vi "Main.vi"(11 "Module Admin":refnum<class "Delacor_lib_QMH_Module Admin.lvclass">) -> ()   [LabVIEW 2023, in "TDMS.lvlib"]
doc: "This template is based off of the Queued Message Handler design pattern and the Queued Message Handler project template that ships with LabVIEW.\n\nThe main difference is that the queue is private to this module and communication between modules is performed via Broadcast and Request events.\n\nRequest events are wrapped in public API methods and are handled in the Event Handling Loop (EHL) of this VI. Any module can register for Broadcast events sent by this module. The EHL generates messages based on user interface actions.\n\nThe Message Handling Loop (MHL) processes messages generated by the EHL, or by other messages. The messages are string values, so new messages can be added easily to the Message Cases case structure in the MHL. Each message cluster can also provide an optional value for Message Data, which is a variant that can be converted to whatever message-specific data is required.\n_____\nBased on DQMH Project Template 7.0.1.1316."
uses:
  TDMS.lvlib
  <vilib>/Delacor/Delacor QMH/Libraries/Module Admin_class/Delacor_lib_QMH_Module Admin.lvclass
  Module Data--cluster.ctl
  Stop Argument--cluster.ctl
  <vilib>/Delacor/Delacor QMH/Libraries/Message Queue_class/Delacor_lib_QMH_Message Queue.lvclass/Delacor_lib_QMH_Message Queue.ctl
  <vilib>/Delacor/Delacor QMH/Libraries/Module Admin_class/Delacor_lib_QMH_Module Admin.lvclass/Delacor_lib_QMH_Module Admin.ctl
  Write Data Argument--cluster.ctl
  Libraries/RT Main/Data Cluster.ctl
  <vilib>/Delacor/Delacor QMH/Libraries/Message Queue_class/Delacor_lib_QMH_Enqueue Message (Single).vi
  <vilib>/Delacor/Delacor QMH/Libraries/Module Admin_class/Delacor_lib_QMH_Get External Launch.vi
  <vilib>/Delacor/Delacor QMH/Libraries/Message Queue_class/Delacor_lib_QMH_Message Queue.lvclass
  Libraries/RT Main/RT Main.lvlib
  <vilib>/WebDAVClient/NI_WebDAV.lvlib
  <vilib>/WebDAVClient/Advanced/Get File.vi
panel:
  out "error out":errorcluster
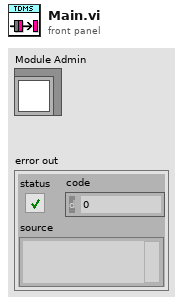
[diagram p1: front panel]
types:
  T1 = typedef "TDMS.lvlib/Request Events--cluster.ctl" = cluster{"Stop Module":refnum<user-event>, "Show Panel":refnum<user-event>, "Hide Panel":refnum<user-event>, "Get Module Execution Status":refnum<user-event>, "Show Diagram":refnum<user-event>, "Create TDMS File":refnum<user-event>, "Close TDMS File":refnum<user-event>, "Write Data":refnum<user-event>, "Private.Write Data to File":refnum<user-event>}
  T2 = typedef "TDMS.lvlib/Module Data--cluster.ctl" = cluster{"Status":string, "Path":path, "tdms file Ref":refnum<k34>}
  T3 = enum32{"invalid lock state", "Not Locked", "Locked (No Password)", "Password-protected"}
  T4 = typedef "TDMS.lvlib/Stop Argument--cluster.ctl" = cluster{"Origin":string, "Exit via Stop Module Req?":bool, "Wait for Module to stop?":bool}
  T5 = typedef "TDMS.lvlib/Write Data Argument--cluster.ctl" = cluster{"Data":T6[]}
  T6 = typedef "RT Main.lvlib/Data Cluster.ctl" = cluster{"Analog Input":dbl[], "Digital Inputs":bool[], "U32":u32[]}
  T7 = enum16{"open", "open or create", "create or replace", "create", "open (read-only)"}
  T8 = typedef "NI_WebDAV.lvlib/SessionHandle.ctl" = refnum<k1>
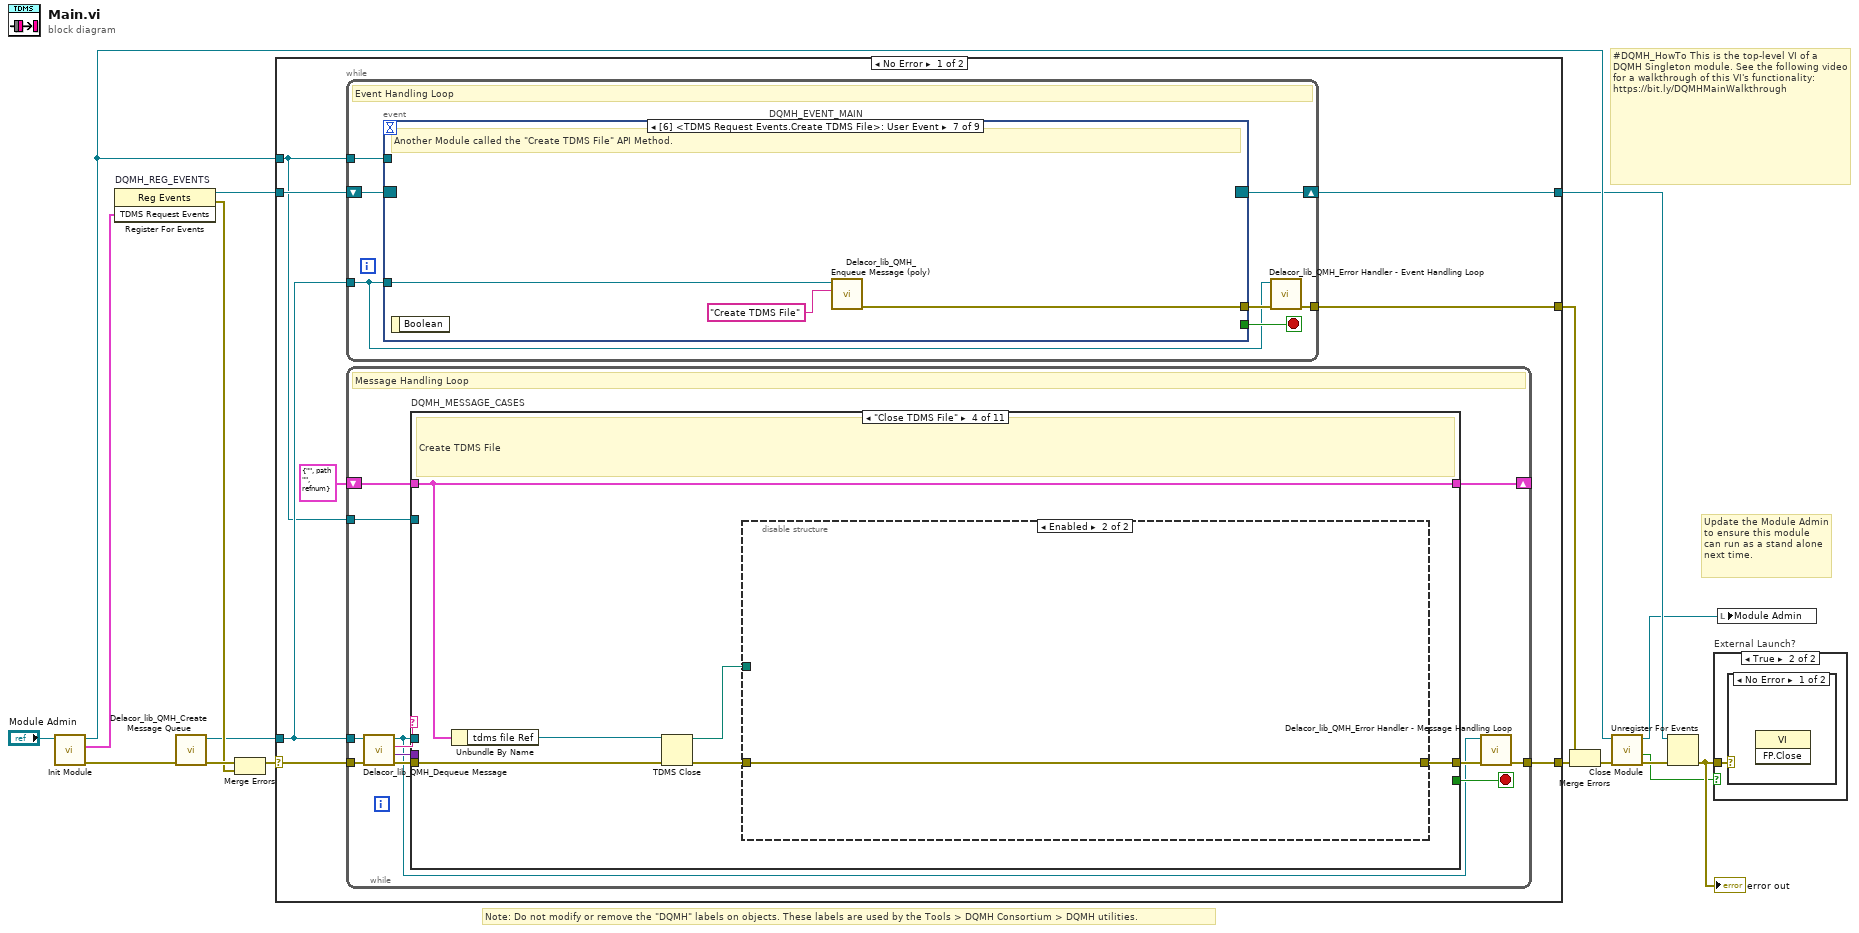
[diagram p0: block diagram]
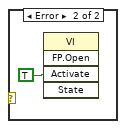
[diagram p3: hidden frame]
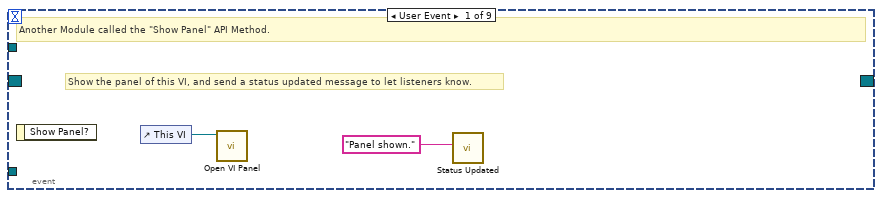
[diagram p4: hidden frame]
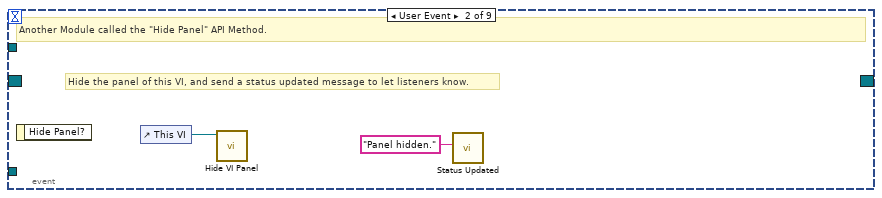
[diagram p5: hidden frame]
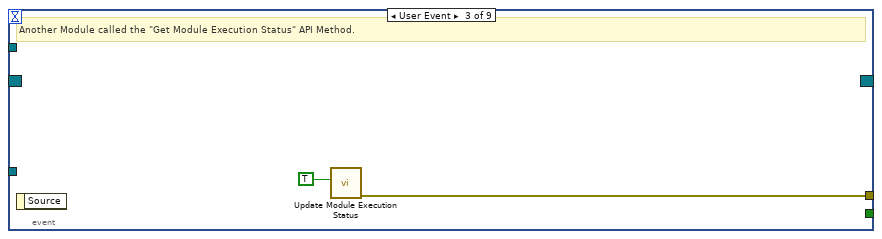
[diagram p6: hidden frame]
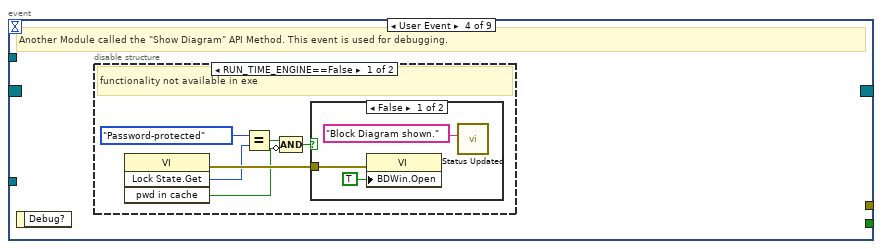
[diagram p7: hidden frame]
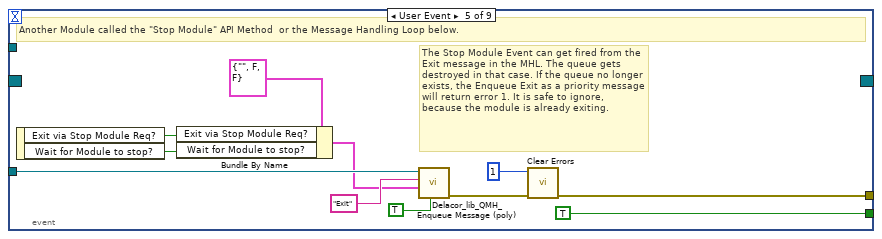
[diagram p10: hidden frame]
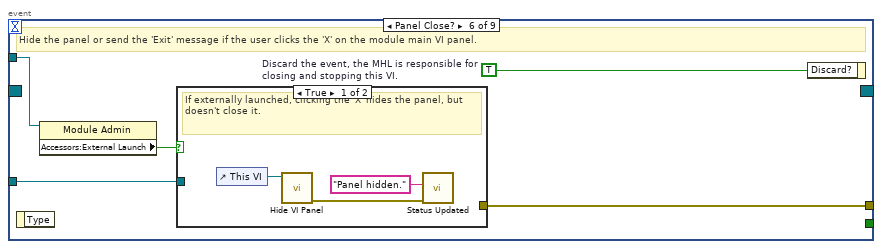
[diagram p11: hidden frame]
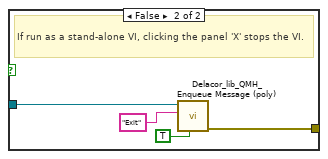
[diagram p12: hidden frame]
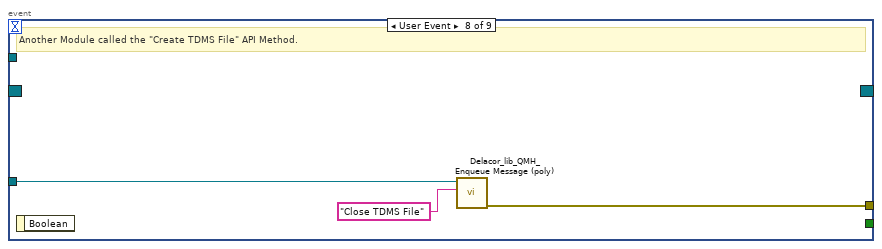
[diagram p13: hidden frame]
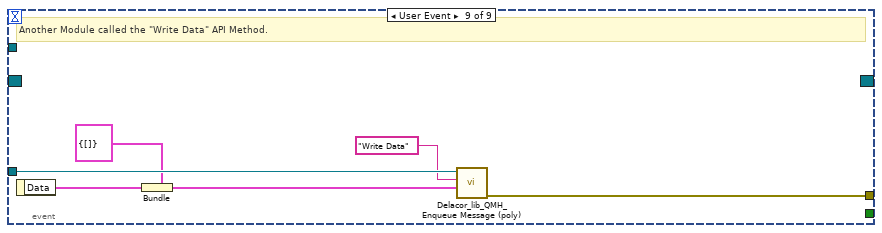
[diagram p14: hidden frame]
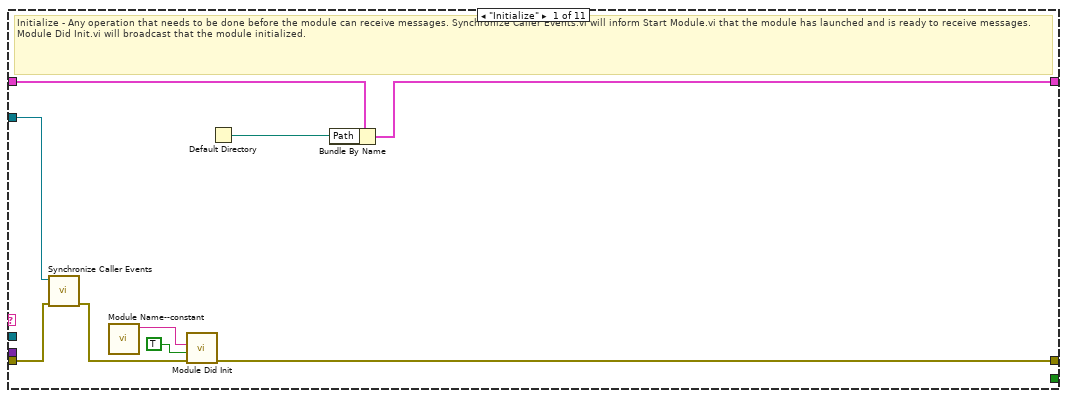
[diagram p15: hidden frame]
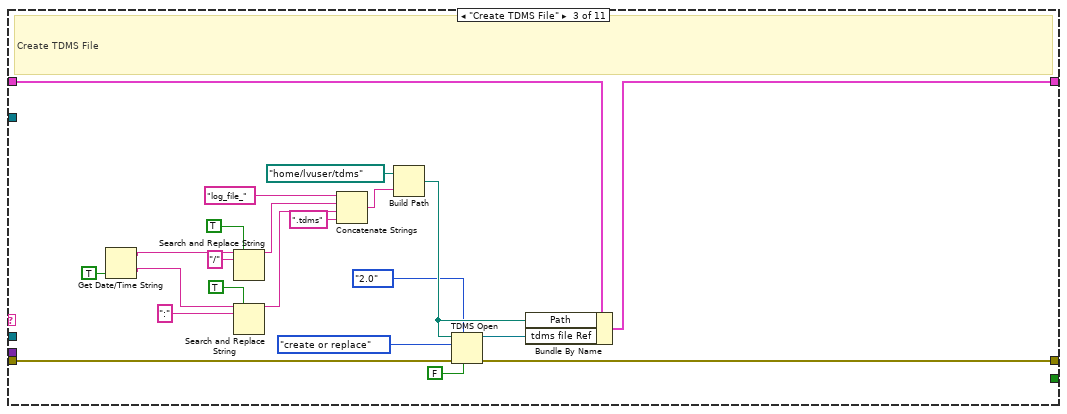
[diagram p17: hidden frame]
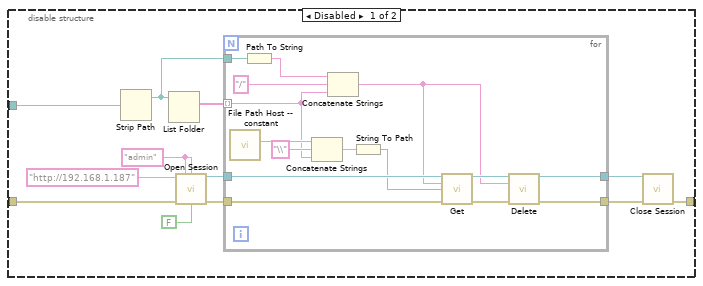
[diagram p18: hidden frame]
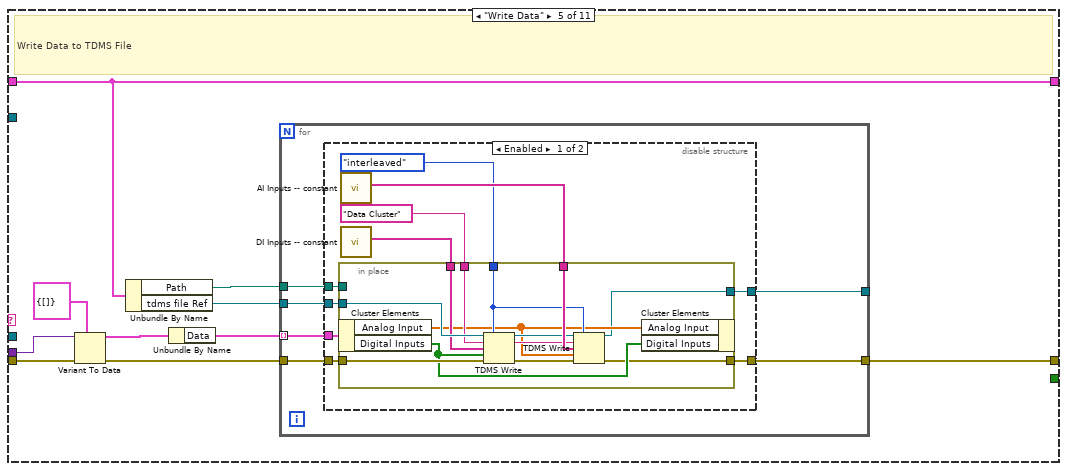
[diagram p19: hidden frame]
diagram:
  # "#DQMH_HowTo This is the top-level VI of a DQMH Singleton module. See the following video for a walkthrough of this VI's functionality: https://bit.ly/DQMHMainWalkthrough"
  # "Note: Do not modify or remove the \"DQMH\" labels on objects. These labels are used by the Tools > DQMH Consortium > DQMH utilities."
  # "Update the Module Admin to ensure this module can run as a stand alone next time."
  n1 = call "Init Module.vi"("Singleton Module Admin in"="Module Admin") -> ("error out"=w16:errorcluster, "TDMS Request Events"=w1:T1, "Singleton Module Admin out"=w8:refnum<class "Delacor_lib_QMH_Module Admin.lvclass">)  [unwired: 8 in]
  n2 = register-events "DQMH_REG_EVENTS"(w1) -> (reference out=w6:refnum<event-registration>, error out=w9:errorcluster)  [unwired: 2 in]
  n3 = call <vilib>:"Delacor_lib_QMH_Create Message Queue.vi"("error in"=w16) -> ("error out"=w11:errorcluster, "Message Queue"=w5:refnum<class "Delacor_lib_QMH_Message Queue.lvclass">)  [unwired: 9 in]
  n4 = Merge Errors(w11, w9) -> (w10:errorcluster)
  n5 = case shown="No Error" w10 {
    selector: w10 -> [w23 w265]
    tunnel: [w25 w264] -> w17
    tunnel: [w22 w263] -> w7
    tunnel: w6 -> [w20 w263]
    tunnel: w5 -> [w19 w258]
    tunnel: [w24 _] -> w14
    tunnel: w8 -> [w18 w259]
    frame No Error {
      n6 = while {
        tunnel: w19 -> [w26]
        shift-right: [w29] -> w22
        shift-left: w20 -> [w30]
        tunnel: [w31] -> w24
        tunnel: w18 -> [w27]
        stop <- w28 stop-if-true
        # "Event Handling Loop"
        n7 = event "DQMH_EVENT_MAIN" shown="[6] <TDMS Request Events.Create TDMS File>: User Event" {
          selector: w30 -> [_ _ _ _ _ _ _ _ _]
          dyn-events: [_ _ _ _ _ _ _ _ _] -> w29
          timeout: _ -> [_ _ _ _ _ _ _ _ _]
          tunnel: [_ _ _ _ TRUE ("Discard?") _ _ _ _] -> w28
          tunnel: w26 -> [_ _ _ _ w54 w61 w73 w76 w82]
          tunnel: [_ _ w38 _ w57 w63 w71 w74 w77] -> w32
          tunnel: w27 -> [_ _ _ _ _ w60 _ _ _]
          event User Event {
            # "Show the panel of this VI, and send a status updated message to let listeners know."
            # "Another Module called the \"Show Panel\" API Method."
            n8 = event-data() -> ()  [unwired: 1 in, 1 out]
            n9 = control-ref of="This VI"() -> (w34:refnum<vi>)
            n10 = call "Open VI Panel.vi"("VI"=w34) -> ()  [unwired: 10 in, 1 out]
            n11 = call "Status Updated.vi"("Status"="Panel shown." ("format string")) -> ()  [unwired: 10 in, 1 out]
          }
          event User Event {
            # "Hide the panel of this VI, and send a status updated message to let listeners know."
            # "Another Module called the \"Hide Panel\" API Method."
            n12 = event-data() -> ()  [unwired: 1 in, 1 out]
            n13 = control-ref of="This VI"() -> (w36:refnum<vi>)
            n14 = call "Hide VI Panel.vi"("VI"=w36) -> ()  [unwired: 10 in, 1 out]
            n15 = call "Status Updated.vi"("Status"="Panel hidden." ("format string")) -> ()  [unwired: 10 in, 1 out]
          }
          event User Event {
            # "Another Module called the \"Get Module Execution Status\" API Method."
            n16 = event-data() -> ()  [unwired: 1 in, 1 out]
            n17 = call "Update Module Execution Status.vi"("Running?"=TRUE) -> ("error out"=w38:errorcluster)  [unwired: 10 in]
          }
          event User Event {
            # "Another Module called the \"Show Diagram\" API Method. This event is used for debugging."
            n18 = event-data() -> ()  [unwired: 1 in, 1 out]
            n19 = disable-structure shown="RUN_TIME_ENGINE==False" {
              frame condition #0 (active) {
                # "functionality not available in exe"
                n20 = invoke on="Invoke Node" class="VI" method="Lock State.Get"() -> (error out=w44:errorcluster, "Get Lock State"=w43:T3, "pwd in cache"=w40:bool)  [unwired: 4 in, 1 out]
                n21 = Equal?(x=T3."Password-protected", y=w43) -> (x = y?=w41:bool)
                n22 = Compound Arithmetic op=AND(w41, invert w40) -> (w39:bool)
                n23 = case shown="False" w39 {
                  tunnel: w44 -> [w47 _]
                  frame False {
                    n24 = property on="Property Node" class="VI"(error in=w47, "BDWin.Open"=TRUE ("Block Diagram Window:Open")) -> ()  [unwired: 1 in, 2 out]
                    n25 = call "Status Updated.vi"("Status"="Block Diagram shown." ("format string")) -> ()  [unwired: 10 in, 1 out]
                  }
                  frame True {
                    # "Password-protected VI, and the password is not in the cache. Do not show the diagram."
                  }
                }
              }
              frame condition #1 {
              }
            }
          }
          event User Event {
            # "The Stop Module Event can get fired from the Exit message in the MHL. The queue gets destroyed in that case. If the queue no longer exists, the Enqueue Exit as a priority message will return error 1. It is safe to ignore, because the module is already exiting."
            # "Another Module called the \"Stop Module\" API Method  or the Message Handling Loop below."
            n26 = event-data() -> ("Exit via Stop Module Req?"=w50:bool, "Wait for Module to stop?"=w49:bool)  [unwired: 1 in]
            n27 = Bundle By Name(cluster=T4 {"Origin"="", "Exit via Stop Module Req?"=FALSE, "Wait for Module to stop?"=FALSE} ("Stop Argument"), "Exit via Stop Module Req?"=w50, "Wait for Module to stop?"=w49) -> (w48:T4)
            n28 = call-poly <vilib>:"Delacor_lib_QMH_Enqueue Message (poly).vi"("Priority Message? (F)"=TRUE, "Message Data"=w48, "Message"="Exit", "Message Queue in"=w54) -> ("error out"=w58:errorcluster)  [unwired: 6 in, 1 out]
            n29 = call <vilib>:"Clear Errors.vi"("error in (no error)"=w58, "specific error code to clear (0: all)"=1) -> ("error out"=w57:errorcluster)  [unwired: 4 in, 1 out]
          }
          event Panel Close? {
            w62 = TRUE  # Discard the event, the MHL is responsible for closing and stopping this VI.
            # "Hide the panel or send the 'Exit' message if the user clicks the 'X' on the module main VI panel."
            n30 = event-data() -> ()  [unwired: 1 in, 1 out]
            n31 = property on="Property Node" class="Module Admin"(reference=w60) -> ("Accessors:External Launch"=w59:bool)  [unwired: 1 in, 2 out]
            n32 = case shown="True" w59 {
              tunnel: w61 -> [_ w69]
              tunnel: [_ w70] -> w63
              frame True {
                # "If externally launched, clicking the 'X' hides the panel, but doesn't close it."
                n33 = control-ref of="This VI"() -> (w66:refnum<vi>)
                n34 = call "Hide VI Panel.vi"("VI"=w66) -> ("error out"=w64:errorcluster)  [unwired: 10 in]
                n35 = call "Status Updated.vi"("error in"=w64, "Status"="Panel hidden." ("format string")) -> ()  [unwired: 9 in, 1 out]
              }
              frame False {
                # "If run as a stand-alone VI, clicking the panel 'X' stops the VI."
                n36 = call-poly <vilib>:"Delacor_lib_QMH_Enqueue Message (poly).vi"("Priority Message? (F)"=TRUE, "Message"="Exit", "Message Queue in"=w69) -> ("error out"=w70:errorcluster)  [unwired: 7 in, 1 out]
              }
            }
            n37 = event-data ("Event Filter Node")("Discard?"=w62) -> ()  [unwired: 1 in, 1 out]
          }
          event User Event {
            # "Another Module called the \"Create TDMS File\" API Method."
            n38 = event-data() -> ()  [unwired: 1 in, 1 out]
            n39 = call-poly <vilib>:"Delacor_lib_QMH_Enqueue Message (poly).vi"("Message"="Create TDMS File", "Message Queue in"=w73) -> ("error out"=w71:errorcluster)  [unwired: 8 in, 1 out]
          }
          event User Event {
            # "Another Module called the \"Create TDMS File\" API Method."
            n40 = event-data() -> ()  [unwired: 1 in, 1 out]
            n41 = call-poly <vilib>:"Delacor_lib_QMH_Enqueue Message (poly).vi"("Message"="Close TDMS File", "Message Queue in"=w76) -> ("error out"=w74:errorcluster)  [unwired: 8 in, 1 out]
          }
          event User Event {
            # "Another Module called the \"Write Data\" API Method."
            n42 = event-data() -> ("Data"=w78:T6[])  [unwired: 1 in]
            n43 = Bundle(cluster=T5 {"Data"=[]} ("Write Data Argument"), "Data"=w78) -> (w79:T5)
            n44 = call-poly <vilib>:"Delacor_lib_QMH_Enqueue Message (poly).vi"("Message Data"=w79, "Message"="Write Data", "Message Queue in"=w82) -> ("error out"=w77:errorcluster)  [unwired: 7 in, 1 out]
          }
        }
        n45 = call-dynamic "Delacor_lib_QMH_Error Handler - Event Handling Loop.vi"("error in"=w32, "Message Queue in"=w26) -> ("dup error in"=w31:errorcluster)  [unwired: 8 in, 1 out]
      }
      n46 = while {
        tunnel: w19 -> [w83]
        shift-right: [w91] -> _
        shift-left: T2 {"Status"="", "Path"=path "", "tdms file Ref"=refnum} ("Data Cluster") -> [w92]
        tunnel: w23 -> [w94]
        tunnel: [w86] -> w25
        tunnel: w18 -> [w87]
        stop <- w90 stop-if-true
        # "Message Handling Loop"
        n47 = call-dynamic "Delacor_lib_QMH_Dequeue Message.vi"("error in"=w94, "Message Queue in"=w83) -> ("error out"=w93:errorcluster, "Message Data"=w88:variant, "Message"=w89:string, "Message Queue out"=w84:refnum<class "Delacor_lib_QMH_Message Queue.lvclass">)  [unwired: 6 in]
        n48 = case "DQMH_MESSAGE_CASES" shown="\"Close TDMS File\"" w89 {
          selector: w89 -> [_ _ _ _ _ _ _ _ _ _ w253]
          tunnel: w84 -> [_ _ _ _ _ _ _ _ w219 w241 _]
          tunnel: w93 -> [w103 w105 w126 w128 w171 w204 w206 w215 w226 w247 w256]
          tunnel: [w98 w105 w127 w130 w162 w203 w206 w214 w222 w242 w257] -> w85
          tunnel: w92 -> [w96 w104 w111 w133 w166 w202 w205 w212 w221 w240 w254]
          tunnel: [w97 w104 w112 w133 w166 w202 w205 w212 w221 w240 w254] -> w91
          tunnel: [_ _ _ _ _ _ _ _ _ w239 _] -> w90
          tunnel: w88 -> [_ _ _ _ w170 _ _ _ w220 w238 _]
          tunnel: w87 -> [w101 _ _ _ _ _ _ _ w218 w233 _]
          frame "Initialize" {
            # "Initialize - Any operation that needs to be done before the module can receive messages. Synchronize Caller Events.vi will inform Start Module.vi that the module has launched and is ready to receive messages. Module Did Init.vi will broadcast that the module initialized."
            n49 = call "Synchronize Caller Events.vi"("error in"=w103, "Singleton Module Admin in"=w101) -> ("error out"=w102:errorcluster)  [unwired: 8 in, 1 out]
            n50 = call "Module Name--constant.vi"() -> ("Module Name"=w99:string)  [unwired: 11 in]
            n51 = call "Module Did Init.vi"("error in"=w102, "Initialized?"=TRUE, "Origin"=w99) -> ("error out"=w98:errorcluster)  [unwired: 8 in]
            n52 = Default Directory() -> (w95:path)
            n53 = Bundle By Name(cluster=w96, "Path"=w95) -> (w97:T2)
          }
          frame "---Module Specific---" {
            # "Separator -- The following cases handle messages specific to this Module."
          }
          frame "Create TDMS File" {
            # "Create TDMS File"
            n54 = Get Date/Time String(want seconds? (F)=TRUE) -> (date string=w118:string, time string=w117:string)  [unwired: 2 in]
            n55 = Search and Replace String(replace all?=TRUE ("replace all? (F)"), input string=w118, search string="/") -> (result string=w116:string)  [unwired: 5 in, 3 out]
            n56 = Search and Replace String(replace all?=TRUE ("replace all? (F)"), input string=w117, search string=":") -> (result string=w115:string)  [unwired: 5 in, 3 out]
            n57 = Concatenate Strings("log_file_", w116, w115, ".tdms" ("string")) -> (w113:string)
            n58 = Build Path(base path=path "/home/lvuser/tdms", name or relative path=w113) -> (appended path=w108:path)
            n59 = TDMS Open(6:FALSE ("disable buffering? (T)"), 7:enum16{"1.0", "2.0"}."2.0" ("file format version (2.0)"), 8:w126, 10:T7."create or replace" ("operation (0:open)"), 11:w108) -> (0:w127:errorcluster, 3:w125:refnum<k34>)  [unwired: 2 in]
            n60 = Bundle By Name(cluster=w111, "Path"=w108, "tdms file Ref"=w125) -> (w112:T2)
          }
          frame "Close TDMS File" {
            # "Create TDMS File"
            n61 = Unbundle By Name(w133) -> ("tdms file Ref"=w129:refnum<k34>)
            n62 = TDMS Close(8:w128, 11:w129) -> (0:w131:errorcluster, 3:w132:path)
            n63 = disable-structure shown="Enabled" {
              disable-tunnel: w132 -> [w145 _]
              disable-tunnel: w131 -> [w143 w161]
              disable-tunnel: [w134 w161] -> w130
              frame Disabled {
                w140 = "admin" ("username")
                n64 = Strip Path(path=w145) -> (stripped path=w137:path)  [unwired: 1 out]
                n65 = List Folder(path=w137) -> (filenames=w144:string[])  [unwired: 3 in, 3 out]
                n66 = call <vilib>:"Open Session.vi"("host uri prefix"="http://192.168.1.187", "username"=w140, "password"=w140, "error in (no error)"=w143, "verify server?"=FALSE) -> ("session handle out"=w141:T8, "error out"=w142:errorcluster)  [unwired: 9 in]
                n67 = for {
                  tunnel: w144 -> [w148] mode=indexing
                  tunnel: w142 -> [w156]
                  tunnel: w141 -> [w160]
                  tunnel: w137 -> [w159]
                  tunnel: [w152] -> w136
                  tunnel: [w151] -> w135
                  n68 = call "File Path Host -- constant.vi"() -> ("File Path Control"=w150:string)  [unwired: 11 in]
                  n69 = Path To String(path=w159) -> (string=w158:string)
                  n70 = Concatenate Strings(w150, "\\" ("string"), w148) -> (w147:string)
                  n71 = Concatenate Strings(w158, "/" ("string"), w148) -> (w154:string)
                  n72 = String To Path(string=w147) -> (path=w146:path)
                  n73 = call-poly <vilib>:"Get.vi"("session handle"=w160, "relative uri"=w154, "local file path"=w146, "error in (no error)"=w156) -> ("session handle out"=w155:T8, "error out"=w153:errorcluster)  [unwired: 9 in, 1 out]
                  n74 = call <vilib>:"Delete.vi"("session handle"=w155, "relative uri"=w154, "error in (no error)"=w153) -> ("session handle out"=w152:T8, "error out"=w151:errorcluster)  [unwired: 11 in]
                }
                n75 = call <vilib>:"Close Session.vi"("session handle"=w136, "error in (no error)"=w135) -> ("error out"=w134:errorcluster)  [unwired: 13 in]
              }
              frame Enabled {
              }
            }
          }
          frame "Write Data" {
            # "Write Data to TDMS File"
            n76 = Variant To Data(error in=w171, type=T5 {"Data"=[]} ("Write Data Argument"), Variant=w170) -> (data=w168:T5, error out=w167:errorcluster)
            n77 = Unbundle By Name(w166) -> ("Path"=w163:path, "tdms file Ref"=w164:refnum<k34>)
            n78 = Unbundle By Name(w168) -> ("Data"=w165:T6[])
            n79 = for {
              tunnel: w167 -> [w177]
              tunnel: w165 -> [w174] mode=indexing
              tunnel: w164 -> [w176]
              tunnel: [w175] -> w162
              tunnel: w163 -> [w173]
              tunnel: [w172] -> _
              n80 = disable-structure shown="Enabled" {
                disable-tunnel: w177 -> [w187 w201]
                disable-tunnel: w176 -> [w186 _]
                disable-tunnel: [w178 w201] -> w175
                disable-tunnel: w174 -> [w181 _]
                disable-tunnel: w173 -> [w180 _]
                disable-tunnel: [w179 _] -> w172
                frame Enabled {
                  n81 = call "AI Inputs -- constant.vi"() -> ("AI Inputs"=w184:string[])  [unwired: 11 in]
                  n82 = call "DI Inputs -- constant.vi"() -> ("DI Inputs"=w185:string[])  [unwired: 11 in]
                  n83 = in-place {
                    in-place-border: w187 -> [w200]
                    in-place-border: w186 -> [w199]
                    in-place-border: w185 -> [w197]
                    in-place-border: w184 -> [w196]
                    in-place-border: enum16{"decimated", "interleaved"}."interleaved" ("data layout (0:decimated)") -> [w194]
                    in-place-border: "Data Cluster" ("group name in (Untitled)") -> [w193]
                    in-place-border: w180 -> [_]
                    in-place-border: [w189] -> w179
                    in-place-border: [w188] -> w178
                    n84 = in-place-cluster #1(w181) -> ("Analog Input"=w191:dbl[], "Digital Inputs"=w190:bool[])
                    n85 = TDMS Write(0:w199, 1:w194, 5:w193, 7:w197, 9:w190, 11:w200) -> (4:w195:refnum<k34>, 6:w192:string, 15:w198:errorcluster)  [unwired: 1 out]
                    n86 = TDMS Write(0:w195, 1:w194, 5:w192, 7:w196, 9:w191, 11:w198) -> (4:w189:refnum<k34>, 15:w188:errorcluster)  [unwired: 2 out]
                    n87 = in-place-cluster #1("Analog Input"=w191, "Digital Inputs"=w190) -> ()  [unwired: 1 out]
                  }
                }
                frame Disabled {
                }
              }
            }
          }
          frame "---Copy This Frame---" {
            # "Duplicate this frame when creating new messages.  Change this comment in the duplicated frame to describe this message."
            n88 = Merge Errors(w204) -> (w203:errorcluster)
          }
          frame "---Exit and Error Handling---" {
            # "Separator - The following cases handle errors and exit messages."
          }
          frame "Simulate MHL Error" {
            # "#DQMH_HowTo The 'Simulate MHL Error' button  illustrates how the MHL handles errors. This event is instructional in nature and can be removed."
            # "Simulate an error occurring at the MHL"
            n89 = call "Module Name--constant.vi"() -> ("Module Name"=w208:string)  [unwired: 11 in]
            n90 = Format Into String(format string="Simulated error originating at Message Handling Loop in %s", w208) -> (resulting string=w209:string)  [unwired: 2 in, 1 out]
            n91 = call <vilib>:"Error Cluster From Error Code.vi"("show call chain? (False)"=TRUE, "error message (\"\")"=w209, "error code (0)"=5001) -> ("error out"=w213:errorcluster)  [unwired: 6 in]
            n92 = Merge Errors(w215, w213) -> (w214:errorcluster)
          }
          frame "Error" {
            # "#CodeRecommended - If the module is running in standalone mode (External Launch = FALSE), this code will pop up an error dialog and call the 'Exit' message if an error occurs. Add more fine-grained error management here."
            # "Error - Check the error message data and respond accordingly. This message is sent by the \"Error Handler\" VIs at the end of each loop in this application."
            n93 = property on="Property Node" class="Module Admin"(reference=w218) -> ("Accessors:External Launch"=w217:bool)  [unwired: 1 in, 2 out]
            n94 = Variant To Data(error in=w226, type=errorcluster {"status"=FALSE, "code"=0, "source"=""} ("error constant"), Variant=w220) -> (data=w216:errorcluster, error out=w224:errorcluster)
            n95 = local write "error out"(w216) -> ()
            n96 = call "Error Reported.vi"("Error"=w216) -> ()  [unwired: 10 in, 1 out]
            n97 = case shown="False" w217 {
              tunnel: [w231 _] -> w223
              tunnel: w219 -> [w229 _]
              tunnel: w216 -> [w230 _]
              frame False {
                n98 = disable-structure shown="Default" {
                  disable-tunnel: w230 -> [w232 _]
                  frame condition #0 (active) {
                    # "If the module is running standalone, then pop up an error dialog and call the \"Exit\" message."
                    n99 = call <vilib>:"Simple Error Handler.vi"("error in (no error)"=w232) -> ()  [unwired: 4 in, 5 out]
                  }
                  frame condition #1 {
                    # "To prevent the Simple Error Handler VI from being loaded (e.g. when deploying to a Real-Time target), add the Conditional Disable Symbol \"DQMH_Disable_SEH\" to your project and set it to TRUE."
                  }
                }
                n100 = call-poly <vilib>:"Delacor_lib_QMH_Enqueue Message (poly).vi"("Priority Message? (F)"=TRUE, "Message"="Exit", "Message Queue in"=w229) -> ("error out"=w231:errorcluster)  [unwired: 7 in, 1 out]
              }
              frame True {
                # "If the module was launched externally, calling the Error Reported broadcast VI is the only action performed by the \"Error\" message. The module's caller can then process the error appropriately."
              }
            }
            n101 = Merge Errors(w224, w223) -> (w222:errorcluster)
          }
          frame "Exit" {
            w237 = 91  # 91: not all Exit messages will have an argument
            w239 = TRUE  # Stop the VI
            # "Release the message queue reference"
            # "Exit - Exit the application."
            n102 = Variant To Data(error in=w247, type=T4 {"Origin"="", "Exit via Stop Module Req?"=FALSE, "Wait for Module to stop?"=FALSE} ("Stop Argument"), Variant=w238) -> (data=w235:T4, error out=w244:errorcluster)
            n103 = call <vilib>:"Clear Errors.vi"("error in (no error)"=w244, "specific error code to clear (0: all)"=w237) -> ("error out"=w246:errorcluster)  [unwired: 4 in, 1 out]
            n104 = control-ref of="This VI"() -> (w234:refnum<vi>)
            n105 = call-dynamic "Delacor_lib_QMH_Release Message Queue.vi"("error in"=w246, "Message Queue"=w241) -> ("error out"=w245:errorcluster)  [unwired: 9 in]
            n106 = call "Handle Exit.vi"("Stop Argument"=w235, "Admin in"=w233, "VI reference"=w234) -> ("error out"=w243:errorcluster)  [unwired: 7 in, 1 out]
            n107 = Merge Errors(w245, w243) -> (w242:errorcluster)
            n108 = call "Error Reported.vi"("Error"=w242) -> ()  [unwired: 10 in, 1 out]
          }
          frame Default {
            # "'Default' case only runs if there is a message that isn't defined in any of the other cases.  Output a programming error."
            n109 = call "Module Name--constant.vi"() -> ("Module Name"=w252:string)  [unwired: 11 in]
            n110 = Format Into String(format string="The invalid message string \"%s\" was received in the Message Handling Loop for module \"%s\".", w253, w252) -> (resulting string=w248:string)  [unwired: 2 in, 1 out]
            n111 = call <vilib>:"Error Cluster From Error Code.vi"("show call chain? (False)"=TRUE, "error message (\"\")"=w248, "error code (0)"=1) -> ("error out"=w255:errorcluster)  [unwired: 6 in]
            n112 = Merge Errors(w256, w255) -> (w257:errorcluster)
          }
        }
        n113 = call-dynamic "Delacor_lib_QMH_Error Handler - Message Handling Loop.vi"("error in"=w85, "Message Queue in"=w84) -> ("dup error in"=w86:errorcluster)  [unwired: 8 in, 1 out]
      }
    }
    frame Error {
      # "Synchronize Caller Events.vi will inform Start Module.vi that the module has launched and will let the code calling Start Module.vi register for broadcasts and would permit the caller receive the broadcast that an error occurred at launch time."
      n114 = call-dynamic "Delacor_lib_QMH_Release Message Queue.vi"("error in"=w265, "Message Queue"=w258) -> ("error out"=w264:errorcluster)  [unwired: 9 in]
      n115 = call "Synchronize Caller Events.vi"("Singleton Module Admin in"=w259) -> ("error out"=w266:errorcluster)  [unwired: 9 in, 1 out]
      n116 = call "Module Name--constant.vi"() -> ("Module Name"=w262:string)  [unwired: 11 in]
      n117 = Format Into String(format string="An error occurred during initialization. %s is no longer running.", w262) -> (resulting string=w260:string)  [unwired: 2 in, 1 out]
      n118 = Merge Errors(w264, w266) -> (w267:errorcluster)
      n119 = call "Error Reported.vi"("Additional Information"=w260, "Error"=w267) -> ()  [unwired: 9 in, 1 out]
    }
  }
  n120 = Merge Errors(w14, w17) -> (w13:errorcluster)
  n121 = call "Close Module.vi"("error in"=w13, "Module Admin in"=w8) -> ("error out"=w15:errorcluster, "External Launch"=w2:bool, "Module Admin out"=w3:refnum<class "Delacor_lib_QMH_Module Admin.lvclass">)  [unwired: 7 in]
  n122 = Unregister For Events(event registration refnum=w7, error in=w15) -> (error out=w12:errorcluster)
  "error out" <- w12
  n123 = case "External Launch?" shown="True" w2 {
    tunnel: w12 -> [_ w268]
    frame False {
    }
    frame True {
      n124 = case shown="No Error" w268 {
        frame No Error {
          n125 = invoke on="Invoke Node" class="VI" method="FP.Close"() -> ()  [unwired: 3 in, 3 out]
        }
        frame Error {
          n126 = invoke on="Invoke Node" class="VI" method="FP.Open"("Activate"=TRUE ("Activate?")) -> ()  [unwired: 4 in, 5 out]
        }
      }
    }
  }
  n127 = local write "Module Admin"(w3) -> ()
